vi "InitEditor.vi"(8 "error in (no error)":errorcluster {"code" format="Error %.0f"}, 10 "VIDoc Settings Path":path, 11 "VIDocEditor in":refnum<class "VIDocEditor.lvclass">) -> (0 "error out":errorcluster {"code" format="Error %.0f"}, 3 "VIDocEditor out":refnum<class "VIDocEditor.lvclass">)   [LabVIEW 2023, in "VIDocEditor.lvclass"]
uses:
  VIDocEditor.lvclass
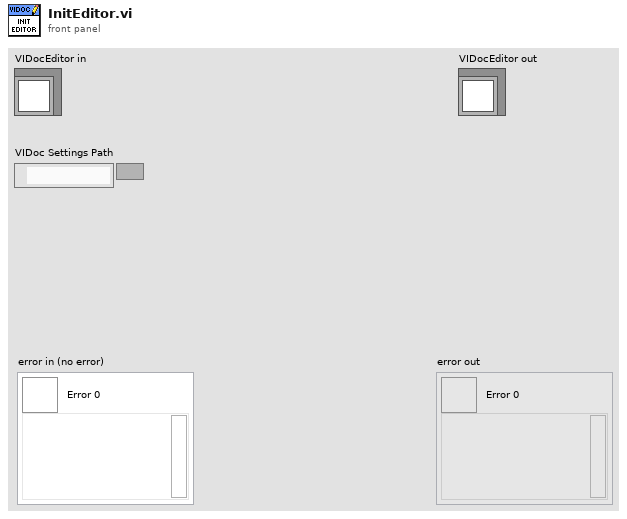
[diagram p1: front panel]
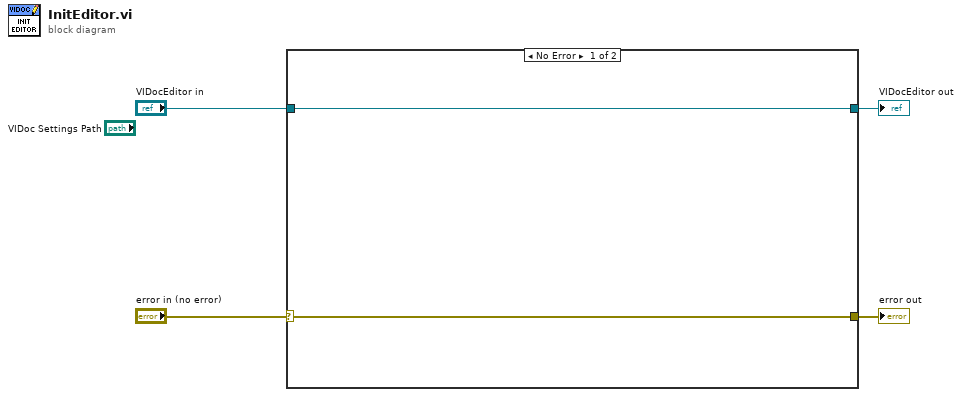
[diagram p0: block diagram]
diagram:
  n1 = case shown="No Error" "error in (no error)" {
    selector: "error in (no error)" -> [w5 w8]
    tunnel: [w5 w8] -> w3
    tunnel: [w6 w7] -> w1
    tunnel: "VIDocEditor in" -> [w6 w7]
    frame No Error {
    }
    frame Error {
    }
  }
  "error out" <- w3
  "VIDocEditor out" <- w1
